vi "TablesToIni.vi"(8 "ErrorArray in":errorcluster[](array[cluster]), 10 "TableRefArray":refnum<vi>[](array[refnum]), 11 "IniFileRef in":T1) -> (0 "ErrorArray out":errorcluster[](array[cluster]), 3 "IniFileRef out":T1)   [LabVIEW 2014, in "Ini_lib.lvlib"]
uses:
  Ini_lib.lvlib
  <vilib>/Utility/config.llb/Config Data RefNum.ctl
  typedefs/clTableData.ctl
  <userlib>/NIST/NISTErrorLib/NISTErrorLib.lvlib
  <vilib>/Utility/config.llb/NI_LVConfig.lvlib
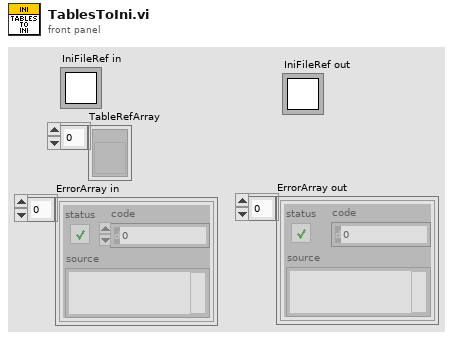
[diagram p1: front panel]
types:
  T1 = typedef "NI_LVConfig.lvlib/Config Data RefNum.ctl" = refnum<k1>
  T2 = typedef "Ini_lib.lvlib/clTableData.ctl" = cluster{"RowHdrs":string[], "ColHdrs":string[], "DefaultParams":string[][]}
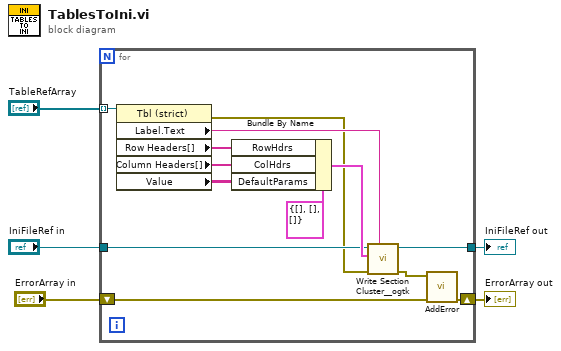
[diagram p0: block diagram]
diagram:
  n1 = for {
    tunnel: "TableRefArray" -> [w18] mode=indexing
    tunnel: "IniFileRef in" -> [w11]
    tunnel: [w10] -> w1
    shift-right: [w9] -> w2
    shift-left: "ErrorArray in" -> [w8]
    n2 = property class="Tbl (strict)"(reference=w18) -> (error out=w6:errorcluster, "Label.Text"=w13:string, "Row Headers[]"=w16:string[], "Column Headers[]"=w15:string[], "Value"=w14:string[][])  [unwired: 1 in, 1 out]
    n3 = Bundle By Name(cluster=T2 {"RowHdrs"=[], "ColHdrs"=[], "DefaultParams"=[]} ("ParamsHdrs"), "RowHdrs"=w16, "ColHdrs"=w15, "DefaultParams"=w14) -> (w12:T2)
    n4 = call <userlib>:"Write Section Cluster__ogtk.vi"("section (optional)"=w13, "error in (no error)"=w6, "Section Formatted Cluster"=w12, "refnum"=w11) -> ("error out"=w7:errorcluster, "dup refnum"=w10:T1)  [unwired: 6 in]
    n5 = call <userlib>:"AddError.vi"("ErrorArray"=w8, "error in (no error)"=w7) -> ("ErrorArray"=w9:errorcluster[])  [unwired: 8 in, 1 out]
  }
  "ErrorArray out" <- w2
  "IniFileRef out" <- w1
